vi "CutData.vi"() -> ()   [LabVIEW 2014]
uses:
  <vilib>/Utility/file.llb/Write To Spreadsheet File (DBL).vi
panel:
  in  "Save":bool
  out "XY Graph":cluster{dbl[], dbl[]}(graph)
  in  "Cut":bool
  in  "End":u32
  in  "Start":u32
  out "Waveform Graph":cluster{"Y":i16[]}[](graph)
  in  "Path":path
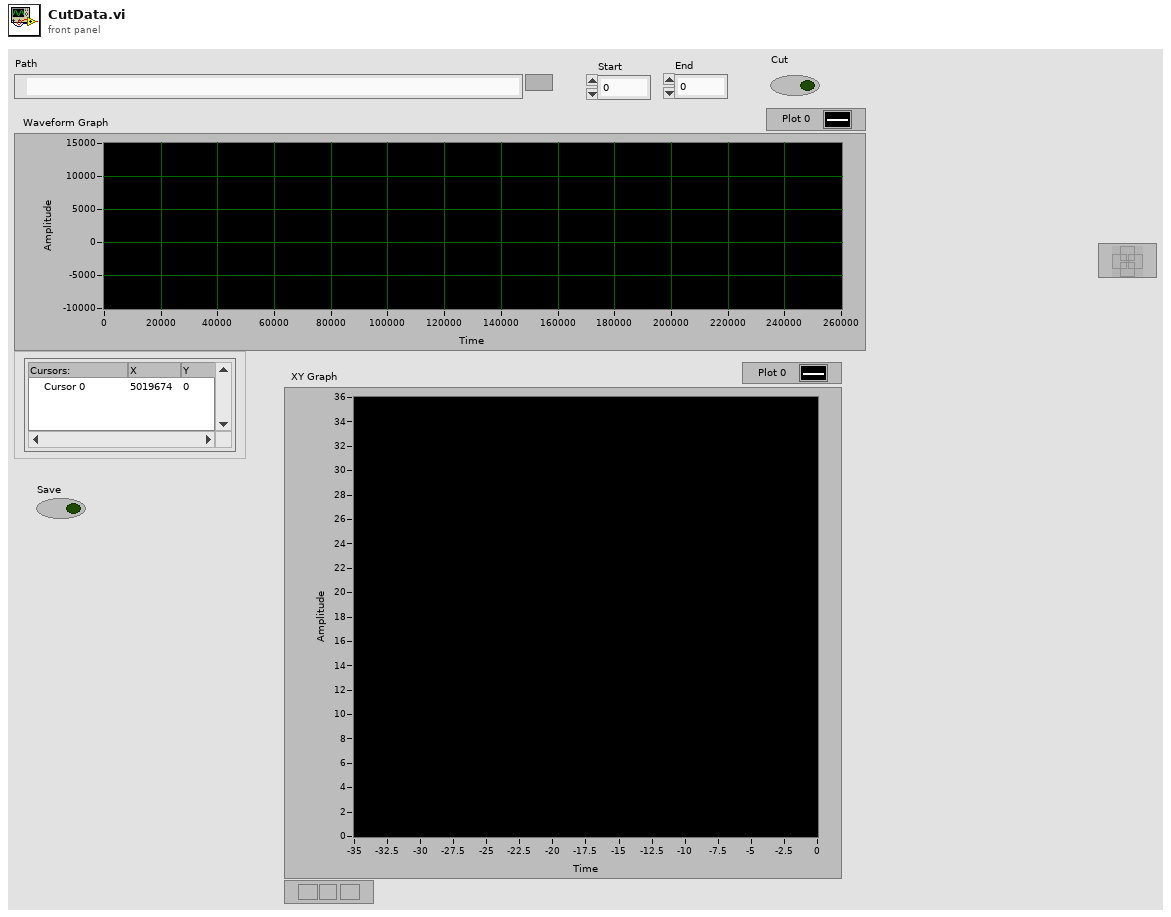
[diagram p1: front panel]
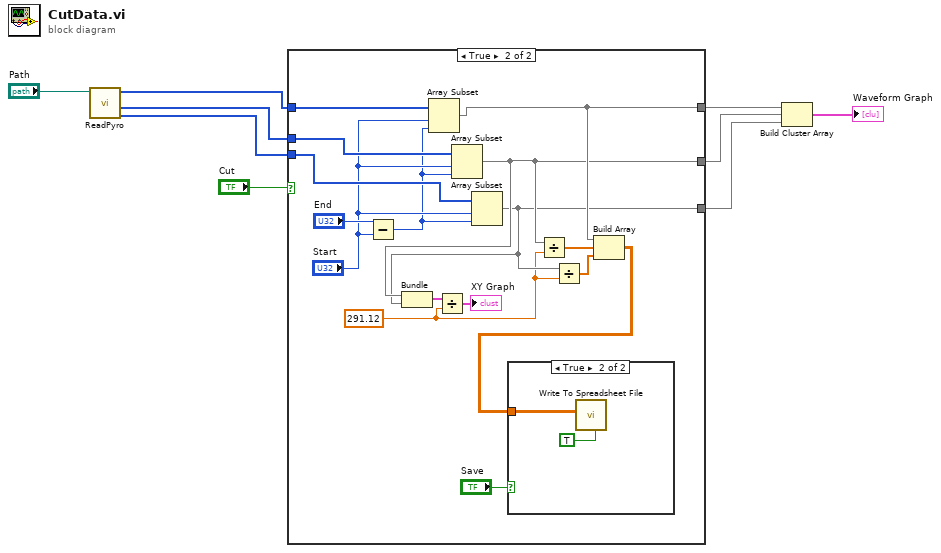
[diagram p0: block diagram]
diagram:
  n1 = call "ReadPyro.vi"("Path"="Path") -> ("Y"=w5:i16[], "X"=w6:i16[], "Pyro1"=w7:i16[])  [unwired: 6 in, 2 out]
  n2 = case shown="True" "Cut" {
    tunnel: w7 -> [w12 w27]
    tunnel: [w12 w18] -> w4
    tunnel: w6 -> [w11 w26]
    tunnel: w5 -> [w10 w25]
    tunnel: [w11 w17] -> w3
    tunnel: [w10 w14] -> w2
    frame False {
    }
    frame True {
      w13 = 291.12
      n3 = Subtract(x="End", y="Start") -> (x-y=w23:u32)
      n4 = Array Subset(array=w27, index="Start", length=w23) -> (w18:i16[])
      n5 = Array Subset(array=w26, index="Start", length=w23) -> (w17:i16[])
      n6 = Array Subset(array=w25, index="Start", length=w23) -> (w14:i16[])
      n7 = Bundle(w17, w14) -> (w22:cluster{i16[], i16[]})  [unwired: 1 in]
      n8 = Divide(x=w22, y=w13) -> (x/y=→"XY Graph":cluster{dbl[], dbl[]})
      n9 = Divide(x=w17, y=w13) -> (x/y=w16:dbl[])
      n10 = Divide(x=w14, y=w13) -> (x/y=w15:dbl[])
      n11 = Build Array(w18, w16, w15) -> (w19:dbl[][])
      n12 = case shown="True" "Save" {
        tunnel: w19 -> [_ w30]
        frame False {
        }
        frame True {
          n13 = call-poly <vilib>:"Write To Spreadsheet File.vi"("transpose? (no:F)"=TRUE, "2D data"=w30) -> ()  [unwired: 6 in, 1 out]
        }
      }
    }
  }
  n14 = Build Cluster Array(w4, w3, w2) -> (→"Waveform Graph":cluster{"Y":i16[]}[])
